vi "Split Ranges.vi"(10 "Parts In":map{string, cluster{"Min":i64, "Max":i64}}(c390), 11 "Expression":string) -> (2 "Parts Out Fail":map{string, cluster{"Min":i64, "Max":i64}}(c390), 3 "Parts Out Pass":map{string, cluster{"Min":i64, "Max":i64}}(c390))   [LabVIEW 2021]
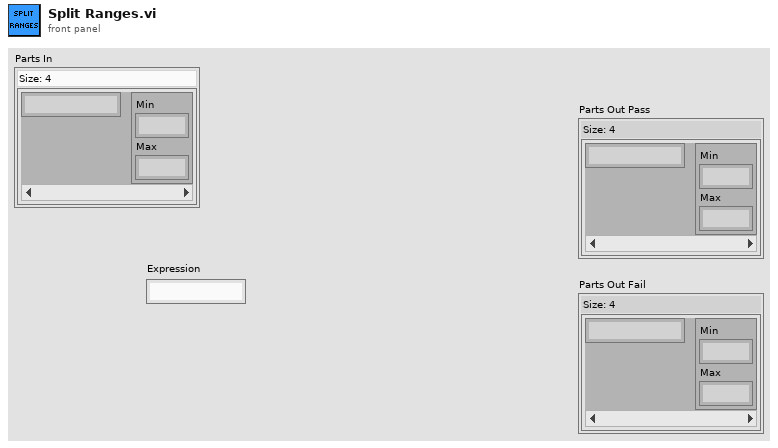
[diagram p1: front panel]
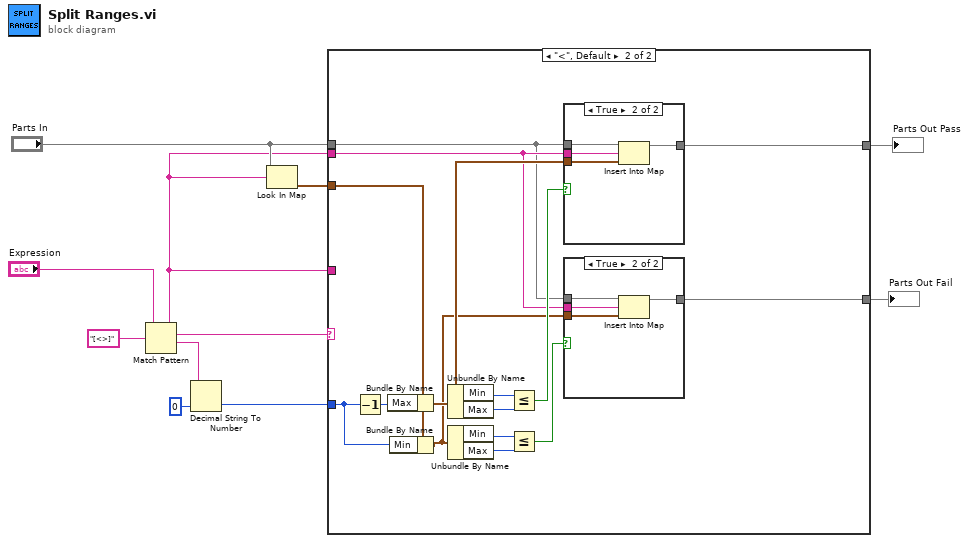
[diagram p0: block diagram]
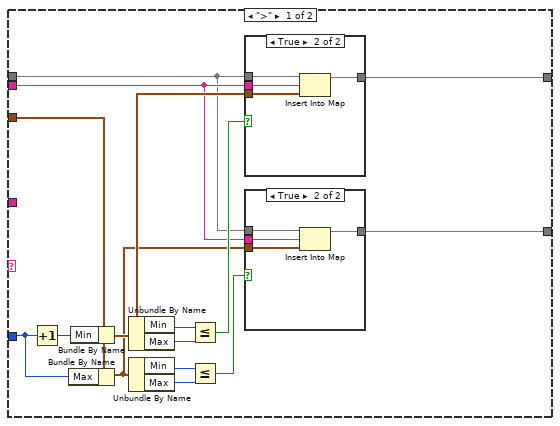
[diagram p2: hidden frame]
diagram:
  n1 = Match Pattern(string="Expression", regular expression="[<>]") -> (before substring=w3:string, match substring=w7:string, after substring=w9:string)  [unwired: 1 in, 1 out]
  n2 = Decimal String To Number(string=w9, default (0L)=i64 0 ("default (0 I32)")) -> (number=w4:i64)  [unwired: 1 in, 1 out]
  n3 = Look In Map(map="Parts In", key=w3) -> (value=w6:cluster{"Min":i64, "Max":i64})  [unwired: 1 in, 1 out]
  n4 = case shown="\"<\", Default" w7 {
    tunnel: w6 -> [w25 w49]
    tunnel: "Parts In" -> [w13 w38]
    tunnel: w3 -> [_ _]
    tunnel: w4 -> [w24 w36]
    tunnel: w3 -> [w14 w39]
    tunnel: [w17 w42] -> w2
    tunnel: [w12 w37] -> w1
    frame ">" {
      n5 = Increment(x=w24) -> (x+1=w26:i64)
      n6 = Bundle By Name(cluster=w25, "Max"=w24) -> (w15:cluster{"Min":i64, "Max":i64})
      n7 = Bundle By Name(cluster=w25, "Min"=w26) -> (w18:cluster{"Min":i64, "Max":i64})
      n8 = Unbundle By Name(w18) -> ("Min"=w23:i64, "Max"=w22:i64)
      n9 = Unbundle By Name(w15) -> ("Min"=w20:i64, "Max"=w21:i64)
      n10 = Less Or Equal?(x=w23, y=w22) -> (x <= y?=w19:bool)
      n11 = Less Or Equal?(x=w20, y=w21) -> (x <= y?=w16:bool)
      n12 = case shown="True" w19 {
        tunnel: w18 -> [_ w32]
        tunnel: w13 -> [_ w34]
        tunnel: w14 -> [_ w33]
        tunnel: [_ w31] -> w17
        frame False {
        }
        frame True {
          n13 = Insert Into Map(map in=w34, key=w33, value=w32) -> (map out=w31:map{string, cluster{"Min":i64, "Max":i64}})  [unwired: 2 out]
        }
      }
      n14 = case shown="True" w16 {
        tunnel: w15 -> [_ w28]
        tunnel: w13 -> [_ w30]
        tunnel: w14 -> [_ w29]
        tunnel: [_ w27] -> w12
        frame False {
        }
        frame True {
          n15 = Insert Into Map(map in=w30, key=w29, value=w28) -> (map out=w27:map{string, cluster{"Min":i64, "Max":i64}})  [unwired: 2 out]
        }
      }
    }
    frame "<", Default {
      n16 = Decrement(x=w36) -> (x-1=w35:i64)
      n17 = Bundle By Name(cluster=w49, "Max"=w35) -> (w43:cluster{"Min":i64, "Max":i64})
      n18 = Bundle By Name(cluster=w49, "Min"=w36) -> (w40:cluster{"Min":i64, "Max":i64})
      n19 = Unbundle By Name(w43) -> ("Min"=w48:i64, "Max"=w47:i64)
      n20 = Unbundle By Name(w40) -> ("Min"=w45:i64, "Max"=w46:i64)
      n21 = Less Or Equal?(x=w48, y=w47) -> (x <= y?=w44:bool)
      n22 = Less Or Equal?(x=w45, y=w46) -> (x <= y?=w41:bool)
      n23 = case shown="True" w44 {
        tunnel: w43 -> [_ w55]
        tunnel: w38 -> [_ w57]
        tunnel: w39 -> [_ w56]
        tunnel: [_ w54] -> w42
        frame False {
        }
        frame True {
          n24 = Insert Into Map(map in=w57, key=w56, value=w55) -> (map out=w54:map{string, cluster{"Min":i64, "Max":i64}})  [unwired: 2 out]
        }
      }
      n25 = case shown="True" w41 {
        tunnel: w40 -> [_ w51]
        tunnel: w38 -> [_ w53]
        tunnel: w39 -> [_ w52]
        tunnel: [_ w50] -> w37
        frame False {
        }
        frame True {
          n26 = Insert Into Map(map in=w53, key=w52, value=w51) -> (map out=w50:map{string, cluster{"Min":i64, "Max":i64}})  [unwired: 2 out]
        }
      }
    }
  }
  "Parts Out Pass" <- w2
  "Parts Out Fail" <- w1
